vi "WSVCAP SHL FPGA LL RFFE FIFO Manager - Transfer.vi"(9 "Word In":u16, 11 "error in (no error)":errorcluster, 13 "Operation":T1) -> (4 "Data Out":u16, 8 "Timed Out":bool, 15 "error out":errorcluster)   [LabVIEW 2012]
uses:
  Type Defs/WSVCAP SHL FIFO Operation Enum.ctl
  <vilib>/rvi/DataTransferAndStorage/Container/XNode/niFpgaContainer.xnode
  <vilib>/rvi/FIFO/Fifo_Resource/nirvififoEmulationWrite.vi
  <vilib>/rvi/FIFO/Fifo_Resource/nirvififoEmulationRead.vi
  <vilib>/rvi/FIFO/Fifo_Resource/nirvififoEmulationGetNumberOfElementsToRead.vi
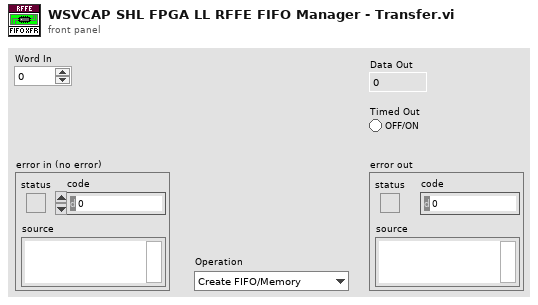
[diagram p1: front panel]
types:
  T1 = typedef "WSVCAP SHL FIFO Operation Enum.ctl" = enum16{"Create FIFO/Memory", "Get Write FIFO Status", "Get Read FIFO Status", "Put Element in Write", "Put Element in Read", "Get Element from Write", "Get Element from Read"}
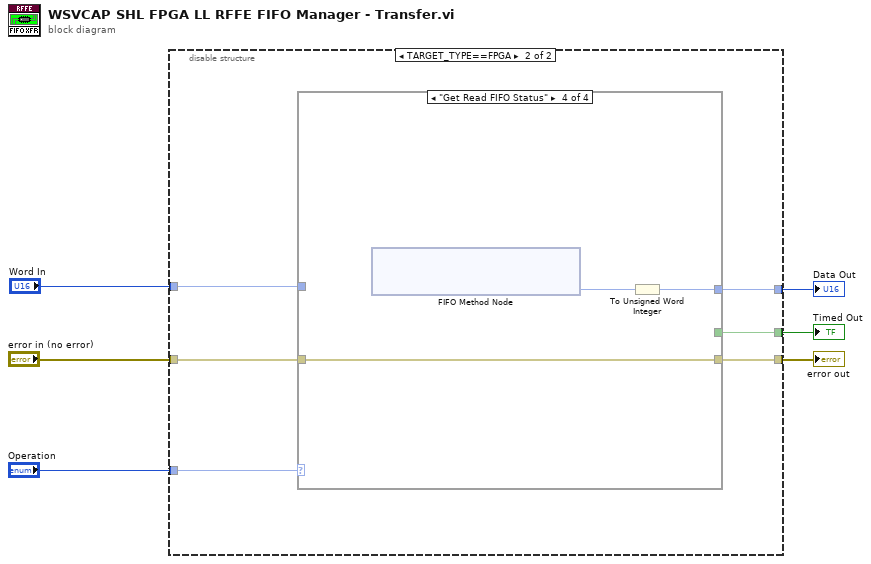
[diagram p0: block diagram]
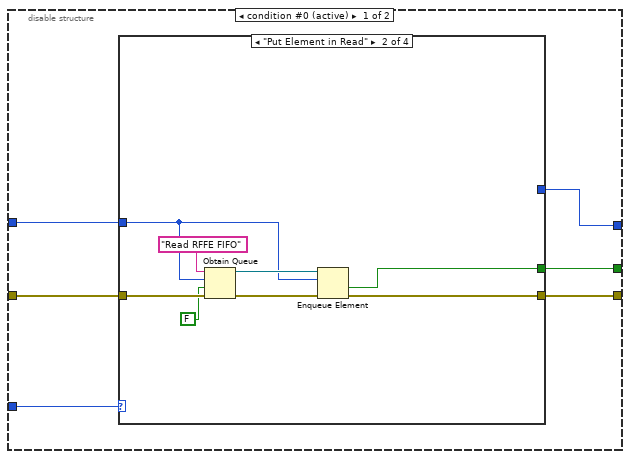
[diagram p2: hidden frame]
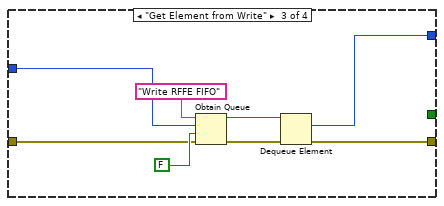
[diagram p4: hidden frame]
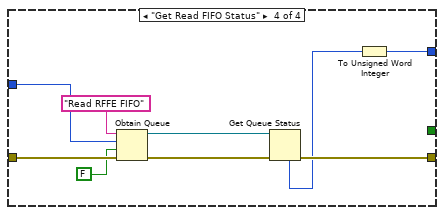
[diagram p5: hidden frame]
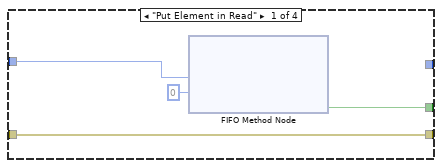
[diagram p6: hidden frame]
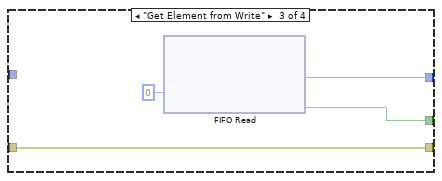
[diagram p8: hidden frame]
diagram:
  n1 = disable-structure shown="TARGET_TYPE==FPGA" {
    disable-tunnel: "Operation" -> [w12 w44]
    disable-tunnel: "error in (no error)" -> [w11 w42]
    disable-tunnel: [w10 w41] -> w4
    disable-tunnel: [w9 w40] -> w1
    disable-tunnel: [w8 w43] -> w3
    disable-tunnel: "Word In" -> [w7 w39]
    frame condition #0 (active) {
      n2 = case shown="\"Put Element in Read\"" w12 {
        tunnel: [w13 w21 w24 w38] -> w10
        tunnel: w11 -> [w13 w19 w25 w37]
        tunnel: [_ _ w22 w30] -> w9
        tunnel: [_ w20 _ _] -> w8
        tunnel: w7 -> [_ w14 w23 w34]
        frame Default {
        }
        frame "Put Element in Read" {
          n3 = Obtain Queue(name (unnamed)="Read RFFE FIFO", element data type=w14, create if not found? (T)=FALSE, error in (no error)=w19) -> (queue out=w17:refnum<queue>, error out=w18:errorcluster)  [unwired: 1 in, 1 out]
          n4 = Enqueue Element(queue=w17, element=w14, error in (no error)=w18) -> (timed out?=w20:bool, error out=w21:errorcluster)  [unwired: 1 in, 1 out]
        }
        frame "Get Element from Write" {
          n5 = Obtain Queue(name (unnamed)="Write RFFE FIFO", element data type=w23, create if not found? (T)=FALSE, error in (no error)=w25) -> (queue out=w27:refnum<queue>, error out=w29:errorcluster)  [unwired: 1 in, 1 out]
          n6 = Dequeue Element(queue=w27, error in (no error)=w29) -> (element=w22:u16, error out=w24:errorcluster)  [unwired: 1 in, 2 out]
        }
        frame "Get Read FIFO Status" {
          n7 = Obtain Queue(name (unnamed)="Read RFFE FIFO", element data type=w34, create if not found? (T)=FALSE, error in (no error)=w37) -> (queue out=w33:refnum<queue>, error out=w32:errorcluster)  [unwired: 1 in, 1 out]
          n8 = Get Queue Status(queue=w33, error in (no error)=w32) -> (error out=w38:errorcluster, # elements in queue=w31:i32)  [unwired: 1 in, 6 out]
          n9 = To Unsigned Word Integer(number=w31) -> (unsigned 16bit integer=w30:u16)
        }
      }
    }
    frame condition #1 {
      n10 = case shown="\"Get Read FIFO Status\"" w44 {
        tunnel: [w47 _ w50 _] -> w43
        tunnel: w42 -> [w48 w49 w53 w54]
        tunnel: [w48 w49 w53 w54] -> w41
        tunnel: [_ _ w52 w55] -> w40
        tunnel: w39 -> [w45 _ _ _]
        frame "Put Element in Read" {
          n11 = xnode ("FIFO Method Node")("Element"=w45, "Timeout"=0) -> ("Timed Out?"=w47:bool)  [unwired: 2 in, 2 out]
        }
        frame Default {
        }
        frame "Get Element from Write" {
          n12 = xnode "FIFO Read"("Timeout"=0) -> ("Element"=w52:u16, "Timed Out?"=w50:bool)  [unwired: 1 in, 1 out]
        }
        frame "Get Read FIFO Status" {
          n13 = xnode ("FIFO Method Node")() -> ("Number of Elements to Read"=w56:u32)  [unwired: 2 in, 2 out]
          n14 = To Unsigned Word Integer(number=w56) -> (unsigned 16bit integer=w55:u16)
        }
      }
    }
  }
  "error out" <- w4
  "Timed Out" <- w3
  "Data Out" <- w1
